vi "StandaloneDemo.vi"() -> ()   [LabVIEW 2013]
uses:
  <vilib>/Platform/browser.llb/Open URL in Default Browser (string).vi
  <vilib>/Heliosphere Research LLC/Advanced Plotting Toolkit/Advanced Plotting Toolkit.lvlib
panel:
  in  "Open URL":bool
  in  "Reset controls":bool
  in  "Run Button":bool
  in  "Ring":u16(ring) items=["Contour Plot", "Filled Contour Plot", "Vector Field", "Streamlines", "Save To Disk", "View Array", "2D Histogram", "1D Histogram", "Transparency", "Line Plot", "Scatter Plot", "Bar Plot", "Polar Plots", "Math Text", "Plot Legend", "Error Bars", "Log Scales", "Tile Plot", "About the Toolkit"]
  in  "stop":bool
  # "Advanced Plotting Toolkit Demo"
  # "Show Demo VI:"
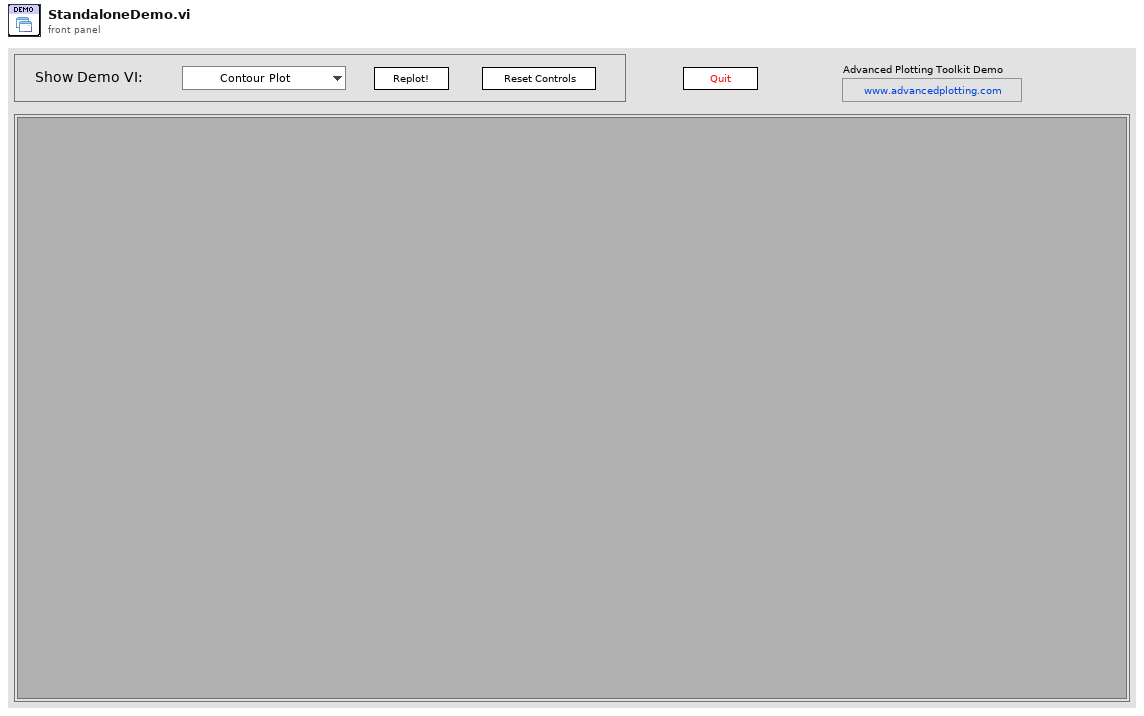
[diagram p1: front panel]
types:
  T1 = enum8{"Enabled", "Disabled", "Disabled and Grayed Out"}
  T2 = enum16{"Always On", "Always Off", "Off While Running"}
  T3 = enum32{"invalid app kind", "Development System", "Run Time System", "Student Edition", "Embedded LabVIEW", "Evaluation", "Custom"}
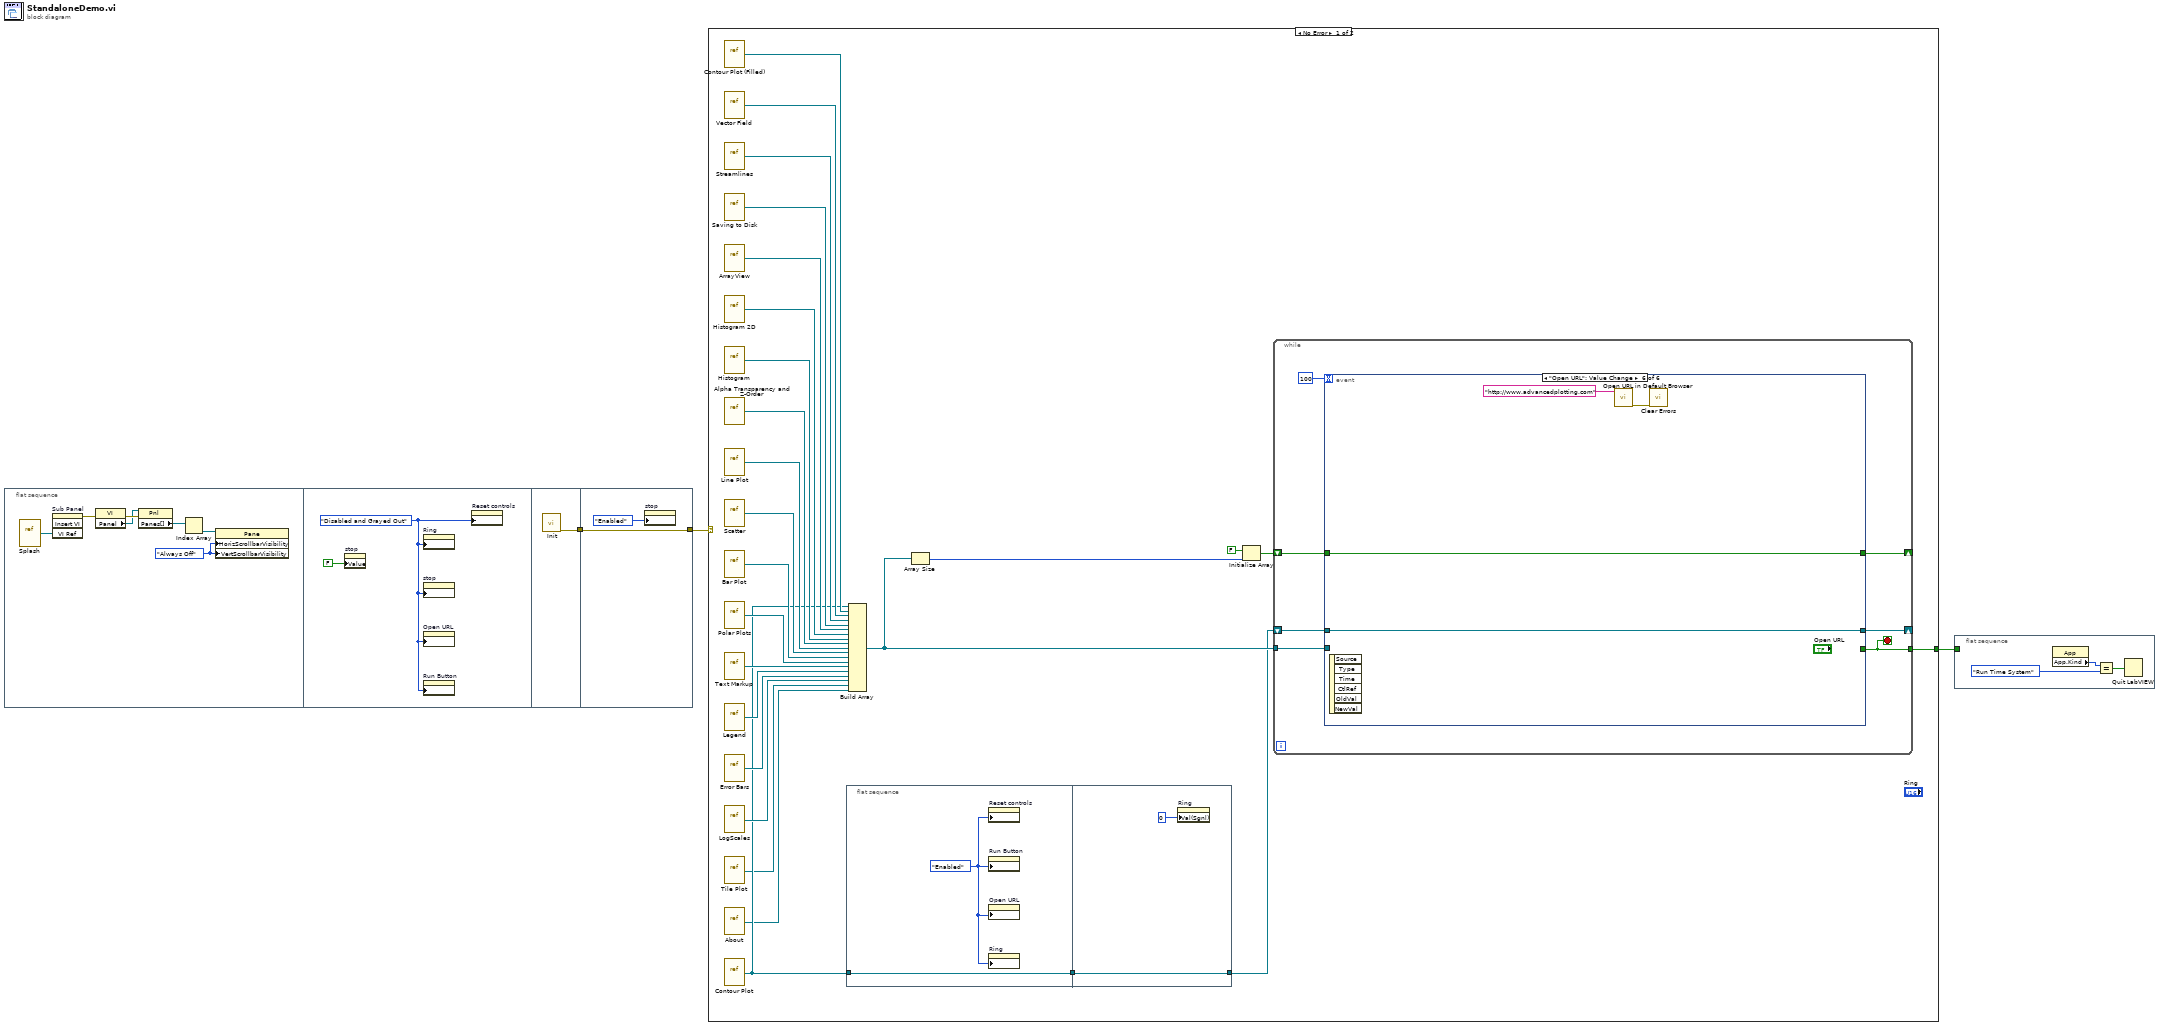
[diagram p0: block diagram]
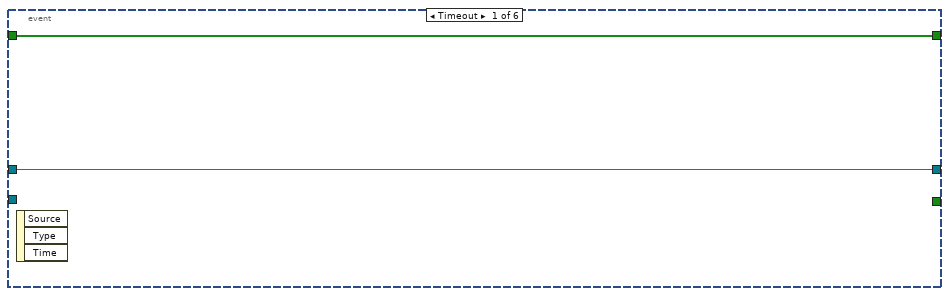
[diagram p2: hidden frame]
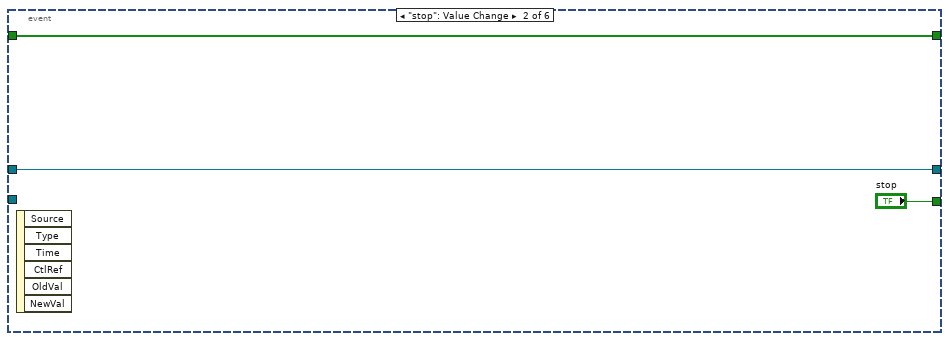
[diagram p3: hidden frame]
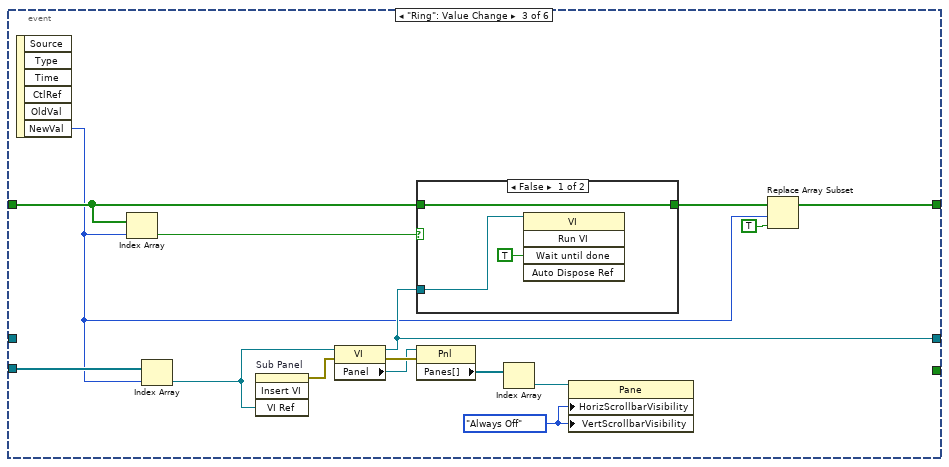
[diagram p4: hidden frame]
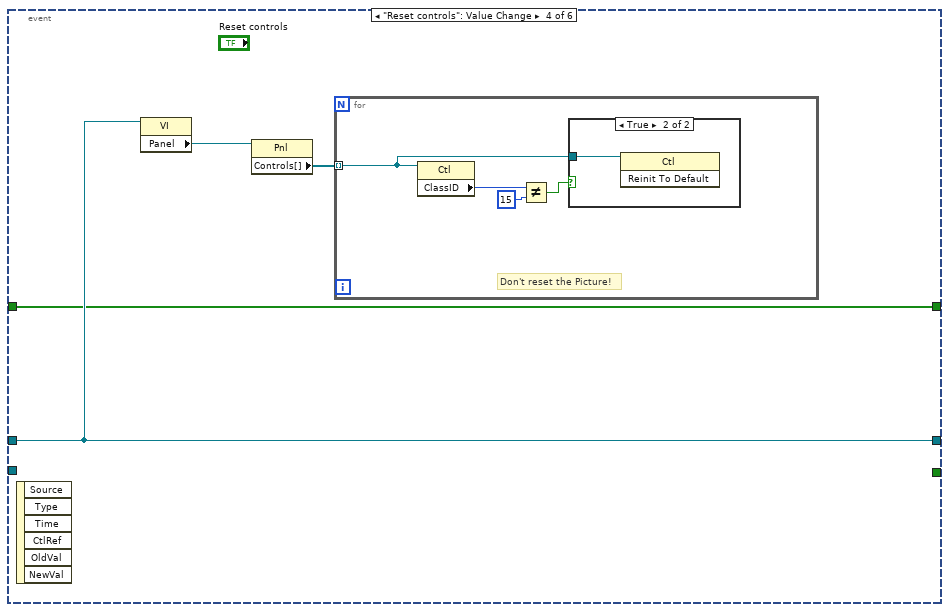
[diagram p6: hidden frame]
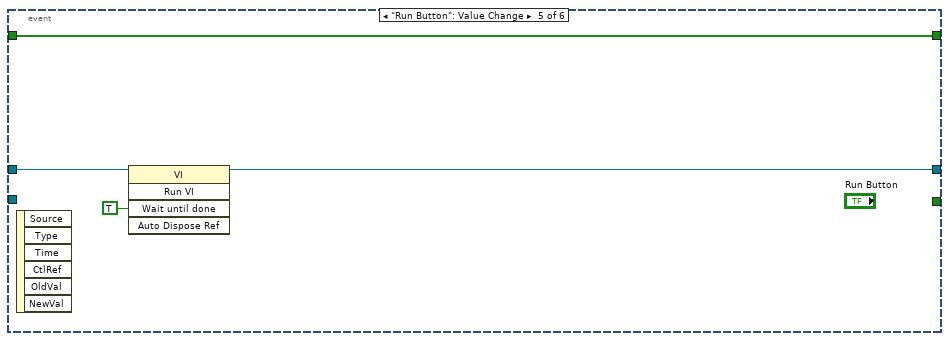
[diagram p8: hidden frame]
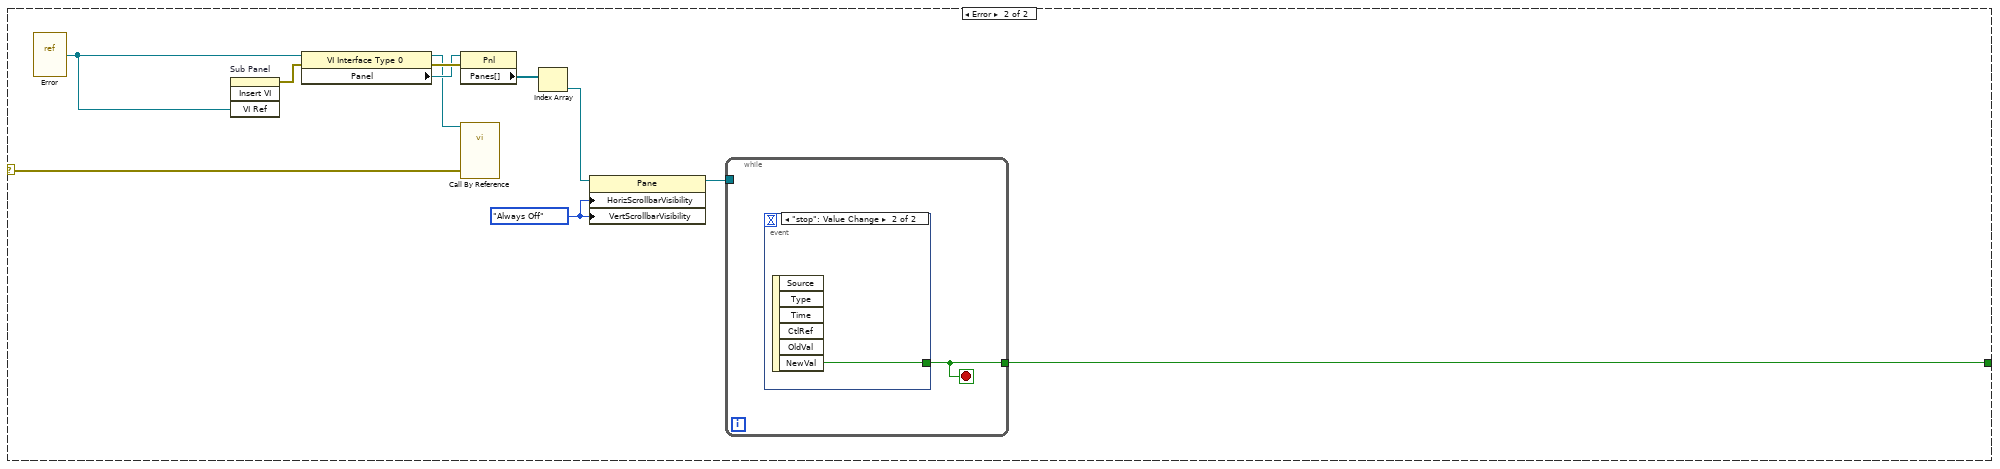
[diagram p9: hidden frame]
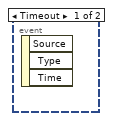
[diagram p10: hidden frame]
diagram:
  n1 = flat-sequence {
    tunnel: [w13] -> w1
    tunnel: [w14] -> w2
    tunnel: w1 -> [w14]
    frame #0 {
      w7 = T2."Always Off" ("Horizontal Scrollbar Visibility")
      n2 = vi-ref "Splash.vi"() -> (w4:refnum<vi>)
      n3 = invoke on="Sub Panel" class="SubPnl" method="Insert VI"("VI Ref"=w4) -> (error out=w10:errorcluster)  [unwired: 3 in, 3 out]
      n4 = property class="VI"(error in=w10) -> (error out=w9:errorcluster, "Panel"=w8:refnum<vi>)  [unwired: 1 in, 1 out]
      n5 = property class="Pnl"(reference=w8, error in=w9) -> ("Panes[]"=w5:refnum<vi>[])  [unwired: 2 out]
      n6 = Index Array(array=w5) -> (element=w6:refnum<vi>)  [unwired: 1 in]
      n7 = property class="Pane"(reference=w6, "HorizScrollbarVisibility"=w7, "VertScrollbarVisibility"=w7) -> ()  [unwired: 1 in, 2 out]
    }
    frame #1 {
      w11 = T1."Disabled and Grayed Out" ("Disabled")
      n8 = property on="stop" class="Bool (strict)"("Value"=FALSE ("stop")) -> ()  [unwired: 2 in, 2 out]
      n9 = property on="Ring" class="Ring (strict)"("DisabledEnum"=w11) -> ()  [unwired: 2 in, 2 out]
      n10 = property on="stop" class="Bool (strict)"("DisabledEnum"=w11) -> ()  [unwired: 2 in, 2 out]
      n11 = property on="Open URL" class="Bool"("DisabledEnum"=w11) -> ()  [unwired: 2 in, 2 out]
      n12 = property on="Run Button" class="Bool"("DisabledEnum"=w11) -> ()  [unwired: 2 in, 2 out]
      n13 = property on="Reset controls" class="Bool"("DisabledEnum"=w11) -> ()  [unwired: 2 in, 2 out]
    }
    frame #2 {
      n14 = call <vilib>:"Init.vi"() -> ("error out"=w13:errorcluster)  [unwired: 11 in]
    }
    frame #3 {
      n15 = property on="stop" class="Bool (strict)"("DisabledEnum"=T1."Enabled" ("Disabled")) -> ()  [unwired: 2 in, 2 out]
    }
  }
  n16 = case shown="No Error" w2 {
    selector: w2 -> [_ w101]
    tunnel: [w41 w102] -> w3
    frame No Error {
      n17 = vi-ref "Contour Plot (Filled).vi"() -> (w40:refnum<vi>)
      n18 = vi-ref "Vector Field.vi"() -> (w39:refnum<vi>)
      n19 = vi-ref "Streamlines.vi"() -> (w38:refnum<vi>)
      n20 = vi-ref "Saving to Disk.vi"() -> (w25:refnum<vi>)
      n21 = vi-ref "ArrayView.vi"() -> (w37:refnum<vi>)
      n22 = vi-ref "Histogram 2D.vi"() -> (w36:refnum<vi>)
      n23 = vi-ref "Histogram.vi"() -> (w35:refnum<vi>)
      n24 = vi-ref "Alpha Transparency and Z-Order.vi"() -> (w34:refnum<vi>)
      n25 = vi-ref "Line Plot.vi"() -> (w33:refnum<vi>)
      n26 = vi-ref "Scatter.vi"() -> (w32:refnum<vi>)
      n27 = vi-ref "Bar Plot.vi"() -> (w31:refnum<vi>)
      n28 = vi-ref "Polar Plots.vi"() -> (w30:refnum<vi>)
      n29 = vi-ref "Text Markup.vi"() -> (w29:refnum<vi>)
      n30 = vi-ref "Legend.vi"() -> (w28:refnum<vi>)
      n31 = vi-ref "Error Bars.vi"() -> (w27:refnum<vi>)
      n32 = vi-ref "LogScales.vi"() -> (w26:refnum<vi>)
      n33 = vi-ref "Tile Plot.vi"() -> (w17:refnum<vi>)
      n34 = vi-ref "About.vi"() -> (w16:refnum<vi>)
      n35 = vi-ref "Contour Plot.vi"() -> (w19:refnum<vi>)
      n36 = flat-sequence {
        tunnel: w19 -> [w43]
        tunnel: [w43] -> w18
        tunnel: [w45] -> w20
        tunnel: w18 -> [w45]
        frame #0 {
          w42 = T1."Enabled" ("Disabled")
          n37 = property on="Reset controls" class="Bool"("DisabledEnum"=w42) -> ()  [unwired: 2 in, 2 out]
          n38 = property on="Run Button" class="Bool"("DisabledEnum"=w42) -> ()  [unwired: 2 in, 2 out]
          n39 = property on="Open URL" class="Bool"("DisabledEnum"=w42) -> ()  [unwired: 2 in, 2 out]
          n40 = property on="Ring" class="Ring (strict)"("DisabledEnum"=w42) -> ()  [unwired: 2 in, 2 out]
        }
        frame #1 {
          n41 = property on="Ring" class="Ring (strict)"("Val(Sgnl)"=u16 0 ("Value (Signaling)")) -> ()  [unwired: 2 in, 2 out]
        }
      }
      n42 = Build Array(w19, w40, w39, w38, w25, w37, w36, w35, w34, w33, w32, w31, w30, w29, w28, w27, w26, w17, w16) -> (w24:refnum<vi>[])
      n43 = Array Size(array=w24) -> (size(s)=w23:i32)
      n44 = Initialize Array(FALSE, w23) -> (w21:bool[])
      n45 = while {
        tunnel: w24 -> [w50]
        shift-right: [w49] -> _
        shift-left: w20 -> [w51]
        tunnel: [w48] -> w41
        shift-right: [w46] -> _
        shift-left: w21 -> [w47]
        stop <- w48 stop-if-true
        n46 = event shown="[5] \"Open URL\": Value Change" {
          selector: _ -> [_ _ _ _ _ _]
          dyn-events: _ -> [_ _ _ _ _ _]
          timeout: 100 -> [_ _ _ _ _ _]
          tunnel: [_ "stop" _ _ _ _] -> w48
          tunnel: w51 -> [w54 w55 _ w78 w88 w93]
          tunnel: w50 -> [_ _ w66 _ _ _]
          tunnel: [w54 w55 w65 w78 w87 w93] -> w49
          tunnel: w47 -> [w53 w56 w62 w77 w86 w92]
          tunnel: [w53 w56 w58 w77 w86 w92] -> w46
          event Timeout {
            n47 = event-data() -> ()  [unwired: 1 in, 3 out]
          }
          event "stop": Value Change {
            n48 = event-data() -> ()  [unwired: 1 in, 6 out]
          }
          event "Ring": Value Change {
            w69 = T2."Always Off" ("Horizontal Scrollbar Visibility")
            n49 = event-data() -> ("NewVal"=w60:u16)  [unwired: 1 in, 5 out]
            n50 = Index Array(array=w62, index=w60) -> (element=w63:bool)
            n51 = Index Array(array=w66, index=w60) -> (element=w64:refnum<vi>)
            n52 = invoke on="Sub Panel" class="SubPanel" method="Insert VI"("VI Ref"=w64) -> (error out=w72:errorcluster)  [unwired: 3 in, 3 out]
            n53 = property class="VI"(reference=w64, error in=w72) -> (reference out=w65:refnum<vi>, error out=w71:errorcluster, "Panel"=w70:refnum<vi>)
            n54 = case shown="False" w63 {
              tunnel: w65 -> [w75 _]
              tunnel: w62 -> [w73 w76]
              tunnel: [w73 w76] -> w61
              frame False {
                n55 = invoke class="VI" method="Run VI"(reference=w75, "Wait until done"=TRUE ("Wait Until Done")) -> ()  [unwired: 3 in, 5 out]
              }
              frame True {
              }
            }
            n56 = property class="Pnl"(reference=w70, error in=w71) -> ("Panes[]"=w67:refnum<vi>[])  [unwired: 2 out]
            n57 = Index Array(array=w67) -> (element=w68:refnum<vi>)  [unwired: 1 in]
            n58 = property class="Pane"(reference=w68, "HorizScrollbarVisibility"=w69, "VertScrollbarVisibility"=w69) -> ()  [unwired: 1 in, 2 out]
            n59 = Replace Array Subset(array=w61, new element=TRUE ("new element/subarray"), index=w60) -> (w58:bool[])
          }
          event "Reset controls": Value Change {
            n60 = event-data() -> ()  [unwired: 1 in, 6 out]
            n61 = property class="VI"(reference=w78) -> ("Panel"=w80:refnum<vi>)  [unwired: 1 in, 2 out]
            n62 = property class="Pnl"(reference=w80) -> ("Controls[]"=w79:refnum<vi>[])  [unwired: 1 in, 2 out]
            n63 = for {
              tunnel: w79 -> [w84] mode=indexing
              # "Don't reset the Picture!"
              n64 = property class="Ctl"(reference=w84) -> ("ClassID"=w83:u32)  [unwired: 1 in, 2 out]
              n65 = Not Equal?(x=w83, y=u32 15) -> (x != y?=w81:bool)
              n66 = case shown="True" w81 {
                tunnel: w84 -> [_ w85]
                frame False {
                }
                frame True {
                  n67 = invoke class="Ctl" method="Reinit To Default"(reference=w85) -> ()  [unwired: 2 in, 3 out]
                }
              }
            }
          }
          event "Run Button": Value Change {
            n68 = event-data() -> ()  [unwired: 1 in, 6 out]
            n69 = invoke class="VI" method="Run VI"(reference=w88, "Wait until done"=TRUE ("Wait Until Done")) -> (reference out=w87:refnum<vi>)  [unwired: 3 in, 4 out]
          }
          event "Open URL": Value Change {
            n70 = event-data() -> ()  [unwired: 1 in, 6 out]
            n71 = call-poly <vilib>:"Open URL in Default Browser.vi"("URL"="http://www.advancedplotting.com") -> ("error out"=w90:errorcluster)  [unwired: 5 in, 1 out]
            n72 = call <vilib>:"Clear Errors.vi"("error in (no error)"=w90) -> ()  [unwired: 6 in, 1 out]
          }
        }
      }
    }
    frame Error {
      w97 = T2."Always Off" ("Horizontal Scrollbar Visibility")
      n73 = vi-ref "Error.vi"() -> (w104:refnum<vi>)
      n74 = invoke on="Sub Panel" class="SubPnl" method="Insert VI"("VI Ref"=w104) -> (error out=w100:errorcluster)  [unwired: 3 in, 3 out]
      n75 = property class="VI Interface Type 0"(reference=w104, error in=w100) -> (reference out=w94:refnum<vi>, error out=w99:errorcluster, "Panel"=w98:refnum<vi>)
      n76 = call-by-ref "?"(reference=w94, "error in (no error)"=w101) -> ()  [unwired: 12 in, 2 out]
      n77 = property class="Pnl"(reference=w98, error in=w99) -> ("Panes[]"=w95:refnum<vi>[])  [unwired: 2 out]
      n78 = Index Array(array=w95) -> (element=w96:refnum<vi>)  [unwired: 1 in]
      n79 = property class="Pane"(reference=w96, "HorizScrollbarVisibility"=w97, "VertScrollbarVisibility"=w97) -> (reference out=w103:refnum<vi>)  [unwired: 1 in, 1 out]
      n80 = while {
        tunnel: w103 -> [_]
        tunnel: [w105] -> w102
        stop <- w105 stop-if-true
        n81 = event shown="[1] \"stop\": Value Change" {
          selector: _ -> [_ _]
          dyn-events: _ -> [_ _]
          timeout: _ -> [_ _]
          tunnel: [_ w106] -> w105
          event Timeout {
            n82 = event-data() -> ()  [unwired: 1 in, 3 out]
          }
          event "stop": Value Change {
            n83 = event-data() -> ("NewVal"=w106:bool)  [unwired: 1 in, 5 out]
          }
        }
      }
    }
  }
  n84 = flat-sequence {
    tunnel: w3 -> [_]
    frame #0 {
      n85 = property class="App"() -> ("App.Kind"=w109:T3)  [unwired: 2 in, 2 out]
      n86 = Equal?(x=w109, y=T3."Run Time System" ("Application:Kind")) -> (x = y?=w107:bool)
      n87 = Quit LabVIEW(quit? (T)=w107) -> ()
    }
  }
